vi "AdsNotification Event Callback.vi"(4 "User Parameter":T1, 5 "Event Data":cluster{"sender":refnum<k24>, "e":refnum<k24>}, 6 "Control Ref":refnum<k24>, 7 "Event Common Data":T3) -> ()   [LabVIEW 2018, in "TwinCAT ADS.lvclass"]
uses:
  TwinCAT ADS.lvclass
  TwinCAT.Ads
  Controls/ADS Notification Callback User Parameter.ctl
  Controls/Notifcation User Event.ctl
  Controls/ADS Notification Event Data.ctl
  Controls/Symbol Information.ctl
  TwinCAT ADS.lvclass/TwinCAT ADS.ctl
  Extensions/Get Symbol Information.vi
  Get From Symbol Map.vi
  Get From Symbol Map Daemon.vi
  Get Symbol Map.vi
  Format String.vi
  Extensions/.Net Symbol Information to G Symbol Information.vi
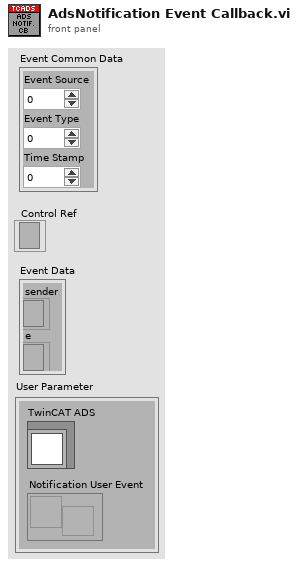
[diagram p1: front panel]
types:
  T1 = typedef "TwinCAT ADS.lvclass/ADS Notification Callback User Parameter.ctl" = cluster{"TwinCAT ADS":refnum<class "TwinCAT ADS.lvclass">, "Notification User Event ":T2}
  T2 = typedef "TwinCAT ADS.lvclass/Notifcation User Event.ctl" = refnum<user-event>
  T3 = cluster{"Event Source":i32, "Event Type":u32, "Time Stamp":u32}
  T4 = typedef "TwinCAT ADS.lvclass/ADS Notification Event Data.ctl" = cluster{"Alias":string, "Symbol Info":T5, "Value":variant}
  T5 = typedef "TwinCAT ADS.lvclass/Symbol Information.ctl" = cluster{"Name":string, "Short Name":string, "Size":i32, "Type Category":i32, "Type Name":string, "Type ID":i32, "Index Group":i64, "Index Offset":i64, "Child Count":i32, "Has Rpc Methods?":bool, "Comment":string}
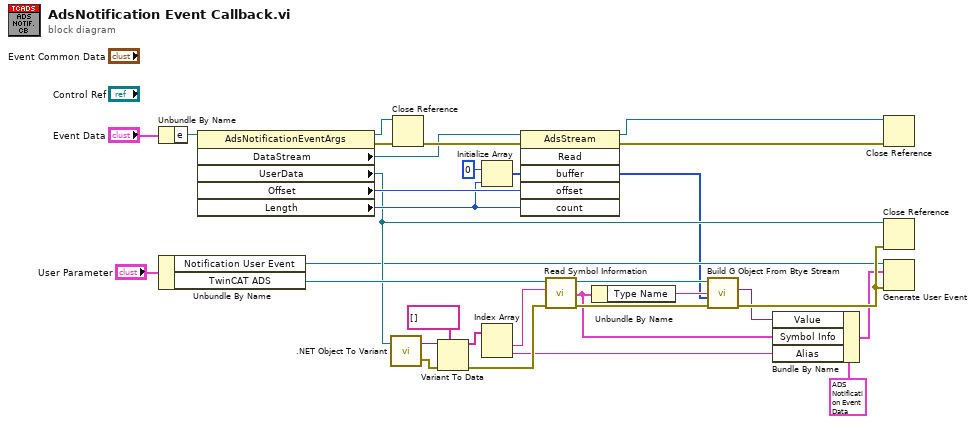
[diagram p0: block diagram]
diagram:
  n1 = Unbundle By Name("Event Data") -> ("e"=w6:refnum<k24>)
  n2 = Unbundle By Name("User Parameter") -> ("Notification User Event"=w4:T2, "TwinCAT ADS"=w14:refnum<class "TwinCAT ADS.lvclass">)
  n3 = property class="AdsNotificationEventArgs"(reference=w6) -> (reference out=w30:refnum<k24>, error out=w31:errorcluster, "DataStream"=w28:refnum<k24>, "UserData"=w8:refnum<k24>, "Offset"=w25:i32, "Length"=w24:i32)  [unwired: 1 in]
  n4 = call <vilib>:".NET Object To Variant.vi"(".NET object"=w8) -> ("error out"=w12:errorcluster, "variant"=w21:variant)  [unwired: 1 in]
  n5 = Close Reference(reference=w30, error in (no error)=w31) -> (error out=w29:errorcluster)
  n6 = Variant To Data(error in=w12, type=string[] [] ("appended array"), Variant=w21) -> (data=w16:string[], error out=w15:errorcluster)
  n7 = Initialize Array(u8 0 ("element"), w24) -> (w26:u8[])
  n8 = Index Array(array=w16) -> (element #1=w13:string, element #2=w9:string)  [unwired: 2 in]
  n9 = invoke class="AdsStream" method="Read"(reference=w28, error in=w29, "buffer"=w26, "offset"=w25, "count"=w24) -> (reference out=w22:refnum<k24>, error out=w23:errorcluster, "buffer"=w1:u8[])  [unwired: 1 in, 3 out]
  n10 = call "Read Symbol Information.vi"("error in (no error)"=w15, "Symbol Name"=w13, "TwinCAT ADS in"=w14) -> ("error out"=w19:errorcluster, "Symbol Information"=w10:T5, "TwinCAT ADS out"=w18:refnum<class "TwinCAT ADS.lvclass">)  [unwired: 6 in]
  n11 = Unbundle By Name(w10) -> ("Type Name"=w17:string)
  n12 = call "Build G Object From Btye Stream.vi"("error in (no error)"=w19, "Byte Stream in"=w1, "Type Name"=w17, "TwinCAT ADS in"=w18) -> ("error out"=w32:errorcluster, "Value"=w2:variant)  [unwired: 4 in, 2 out]
  n13 = Bundle By Name(cluster=T4 {"Alias"="", "Symbol Info"={"Name"="", "Short Name"="", "Size"=0, "Type Category"=0, "Type Name"="", "Type ID"=0, "Index Group"=0, "Index Offset"=0, "Child Count"=0, "Has Rpc Methods?"=FALSE, "Comment"=""}, "Value"=variant} ("event data"), "Value"=w2, "Symbol Info"=w10, "Alias"=w9) -> (w3:T4)
  n14 = Close Reference(reference=w22, error in (no error)=w23) -> ()  [unwired: 1 out]
  n15 = Close Reference(reference=w8, error in (no error)=w32) -> ()  [unwired: 1 out]
  n16 = Generate User Event(user event=w4, event data cluster=w3, error in=w32) -> ()  [unwired: 1 in, 2 out]
